vi "VISA_ReadAndSave_8CHparalelos.vi"() -> ()   [LabVIEW 2019]
uses:
  813f916b-c519-439e-9418-14bd48b6d342.vi
  <vilib>/Instr/_visa.llb/VISA Configure Serial Port (Instr).vi
  <vilib>/Analysis/Matrix/Comparison/Not Equal/Not Equal.vi
  <vilib>/Analysis/Matrix/Comparison/Not Equal/Not Equal - RM,RM.vi
panel:
  out "loop delay":dbl format="%.2f"
  out "Plot 7":dbl[](graph)
  out "Plot 6":dbl[](graph)
  out "Plot 5":dbl[](graph)
  out "Plot 4":dbl[](graph)
  out "Plot 3":dbl[](graph)
  out "Plot 2":dbl[](graph)
  out "error file":errorcluster
  in  "file name":string
  out "Plot 1":dbl[](graph)
  out "Plot 0":dbl[](graph)
  out "Status Read":errorcluster
  out "Buffer Array":dbl[](array[numeric])
  out "Read Buffer":string
  out "Status Serial":errorcluster
  in  "Stop Read":bool
  in  "Start Read":bool
  in  "baud rate (115200)":u32=115200 caption="baud rate (9600)"
  in  "data bits (8)":u8=8 min=5 max=8 step=1
  in  "VISA resource name":refnum<visa-resource-name>="COM3"
  # "Controle de Salvamento"
  # "Log de Erros"
  # "Conversão Para Inteiro"
  # "Resultado da Leitura"
  # "Controle da porta Serial USB"
  # "Controle da Leitura"
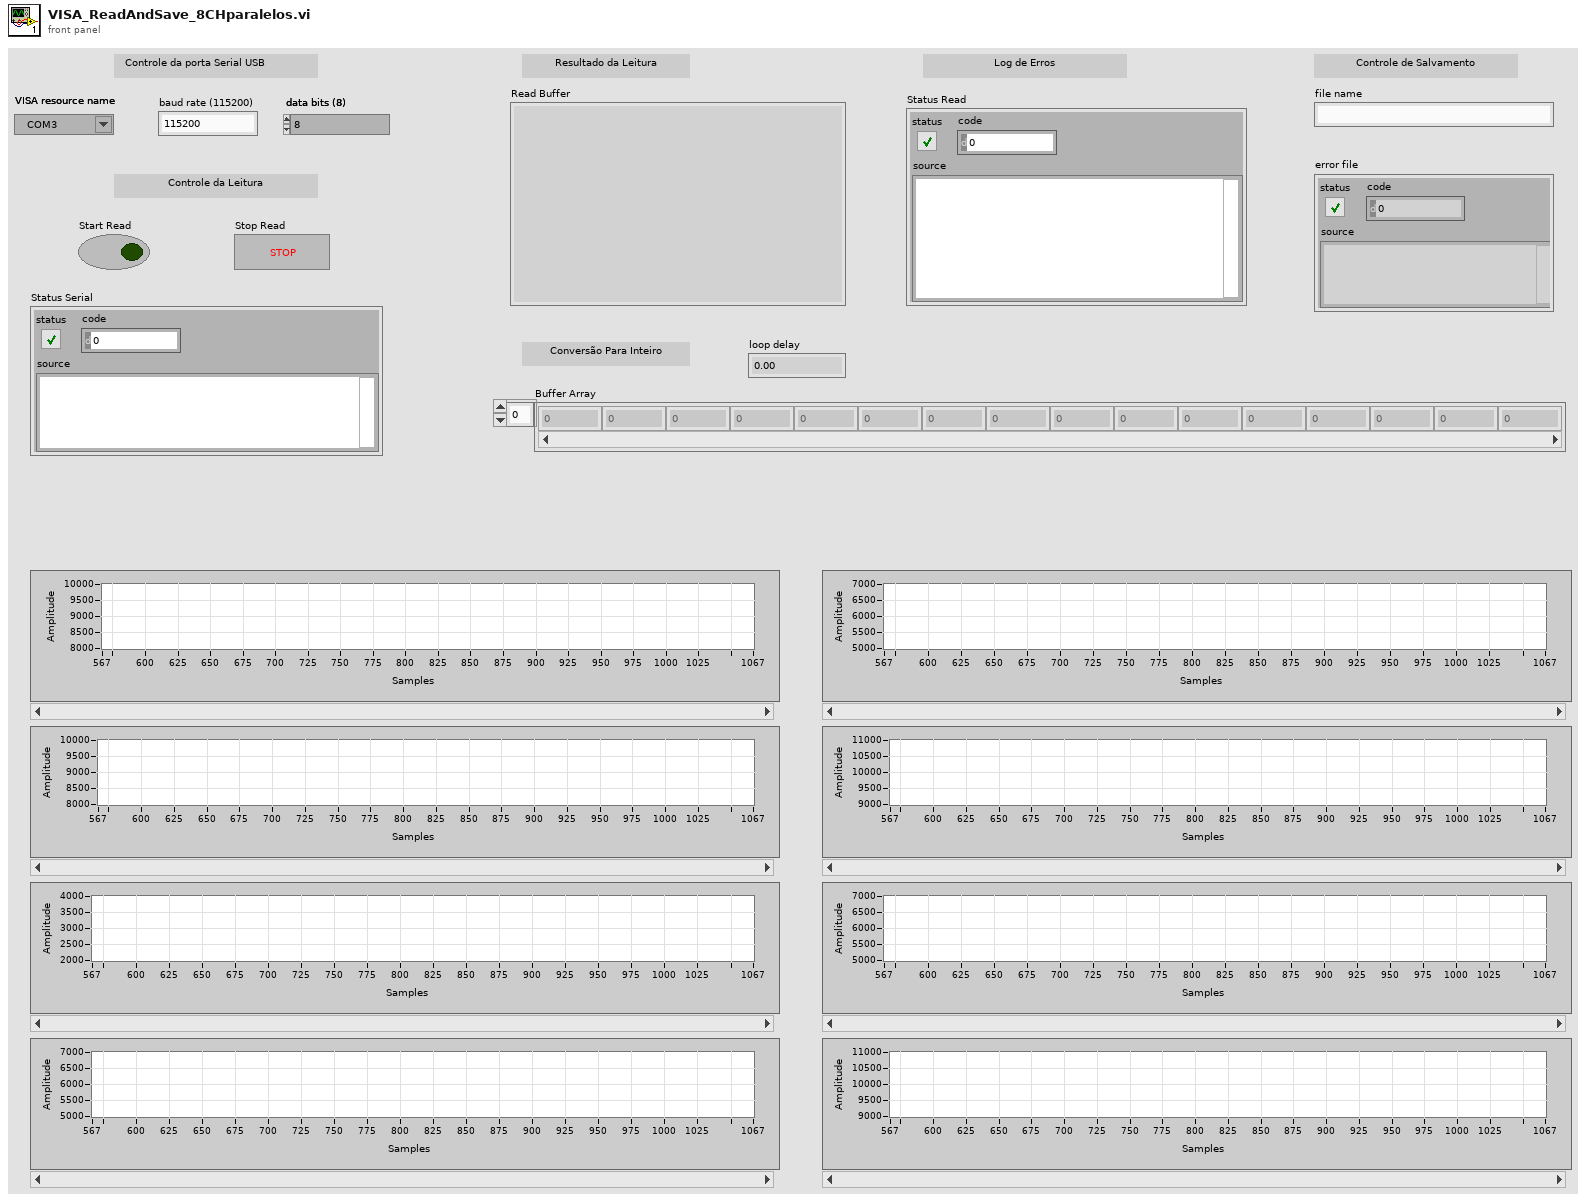
[diagram p1: front panel]
types:
  T1 = typedef "NI_Matrix.lvlib/RealMatrix.ctl" = dbl[][]
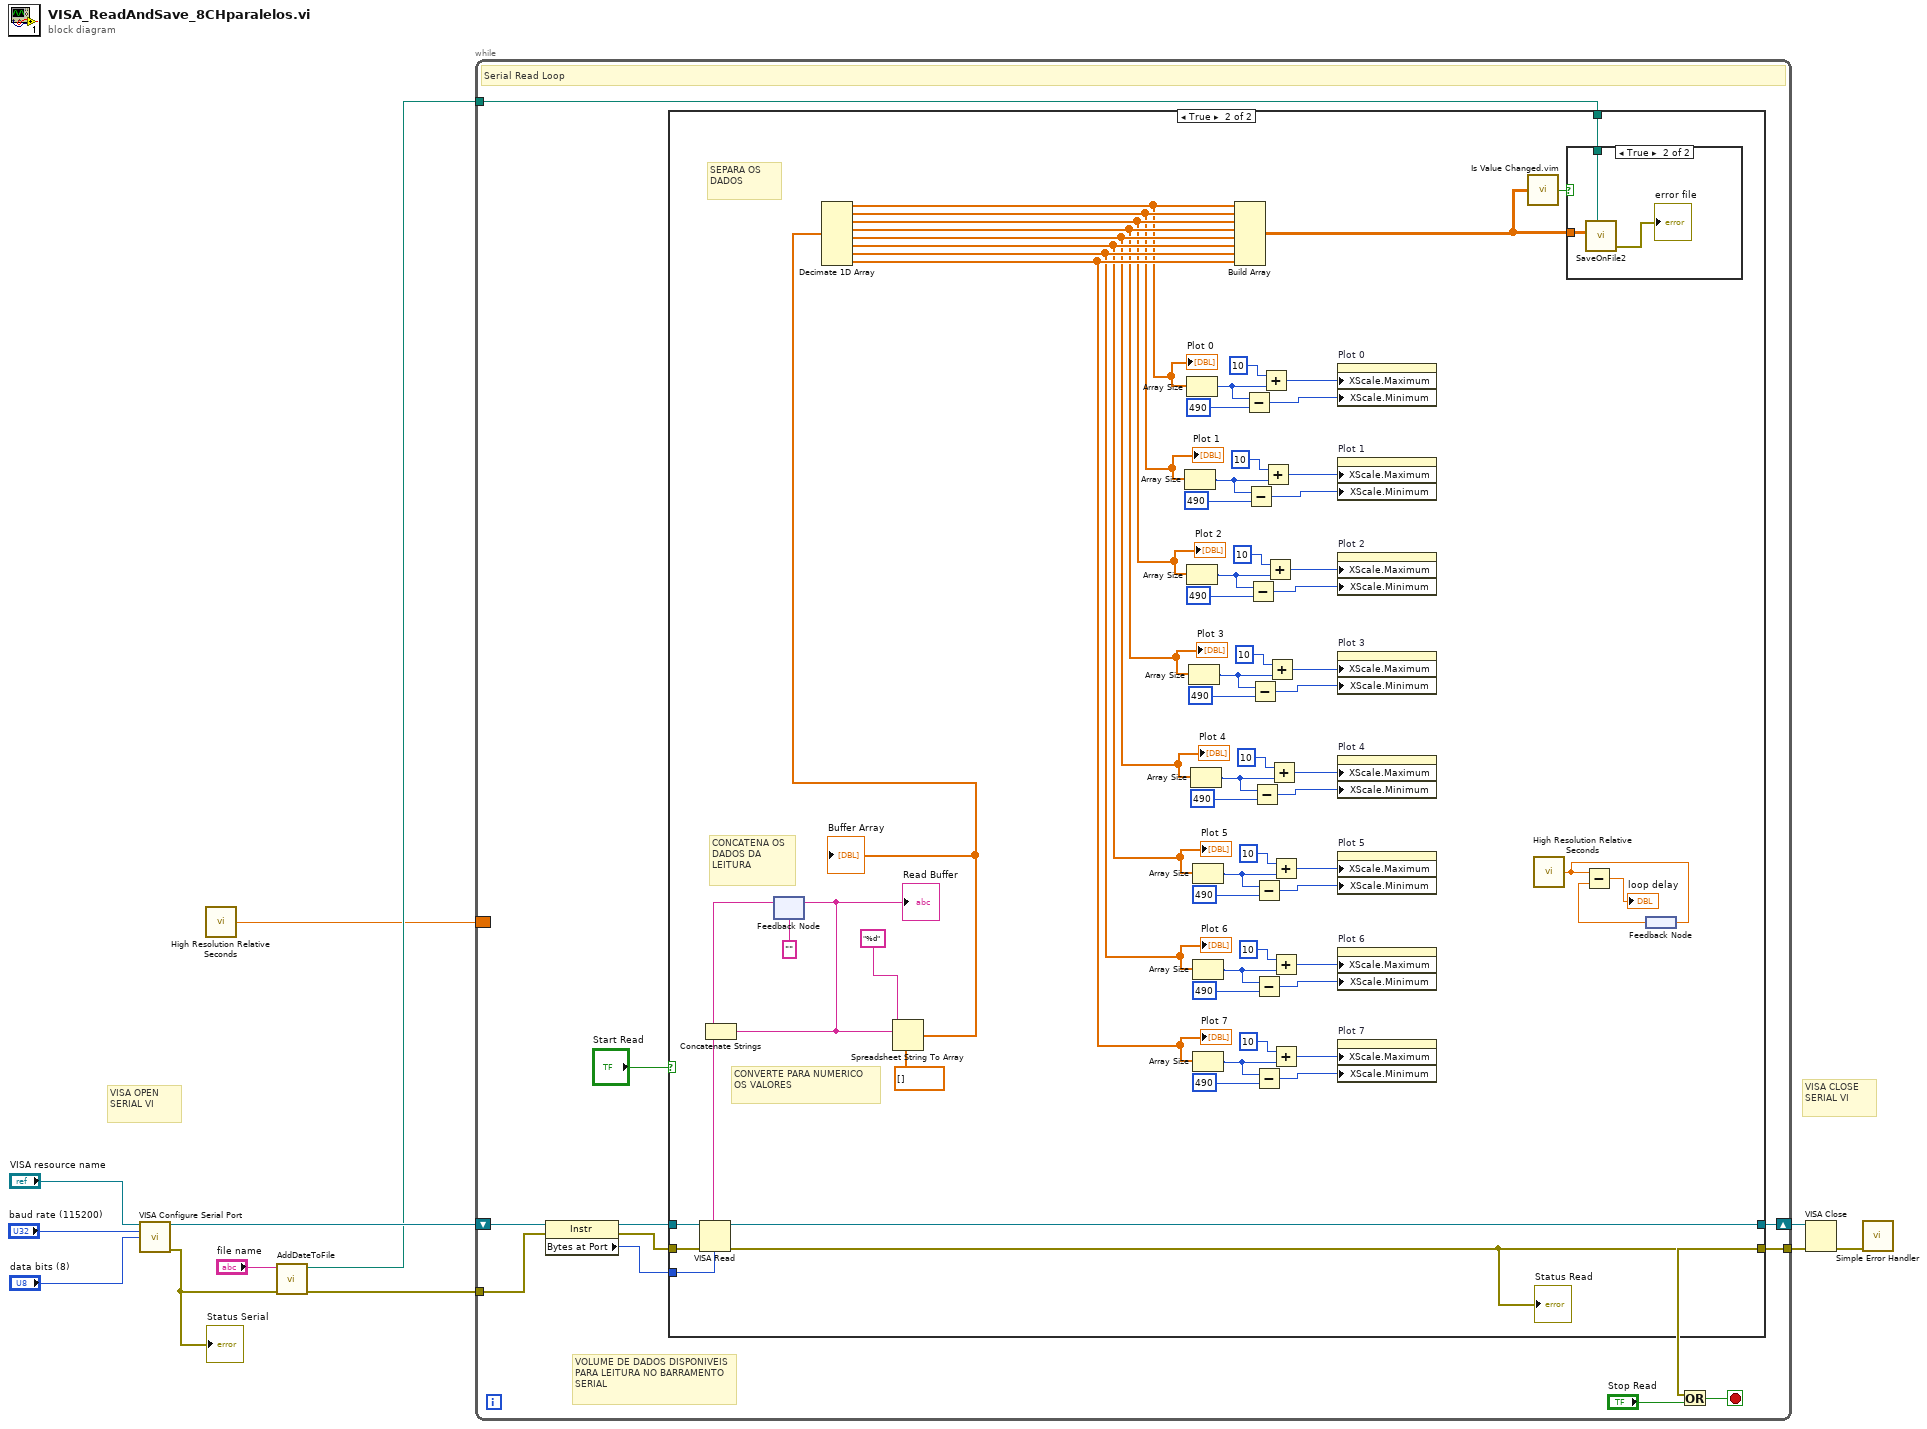
[diagram p0: block diagram]
diagram:
  # "VISA OPEN SERIAL VI"
  # "VISA CLOSE SERIAL VI"
  n1 = call-poly "VISA Configure Serial Port"("VISA resource name"="VISA resource name", "baud rate (9600)"="baud rate (115200)", "data bits (8)"="data bits (8)") -> ("VISA resource name out"=w10:refnum<visa-resource-name>, "error out"=w3:errorcluster)  [unwired: 11 in]
  "Status Serial" <- w3
  n2 = call <vilib>:"High Resolution Relative Seconds.vi"() -> ("relative seconds"=w1:dbl)
  n3 = call "AddDateToFile.vi"("error in (no error)"=w3, "file name"="file name") -> ("error out"=w4:errorcluster, "new file path (Not A Path if cancelled)"=w2:path)  [unwired: 8 in]
  n4 = while {
    tunnel: w4 -> [w14]
    tunnel: [w21] -> w11
    shift-right: [w20] -> w9
    shift-left: w10 -> [w18]
    tunnel: w2 -> [w13]
    border: w1 -> [_]
    stop <- w19 stop-if-true
    # "VOLUME DE DADOS DISPONIVEIS PARA LEITURA NO BARRAMENTO SERIAL"
    # "Serial Read Loop"
    n5 = property class="Instr"(reference=w18, error in=w14) -> (reference out=w15:refnum<visa-resource-name>, error out=w16:errorcluster, "Bytes at Port"=w17:u32)
    n6 = case shown="True" "Start Read" {
      tunnel: [w24 w91] -> w21
      tunnel: [w25 w89] -> w20
      tunnel: w17 -> [_ w85]
      tunnel: w15 -> [w25 w84]
      tunnel: w16 -> [w24 w83]
      tunnel: w13 -> [_ w75]
      frame False {
        # "OS DADOS SÃO ACUMULADOS NO BUFFER ESPERANDO A PERMISSÃO PARA SER LIDOS"
      }
      frame True {
        # "SEPARA OS DADOS"
        # "CONVERTE PARA NUMERICO OS VALORES"
        # "CONCATENA OS DADOS DA LEITURA"
        n7 = VISA Read(VISA resource name=w84, byte count=w85, error in (no error)=w83) -> (VISA resource name out=w89:refnum<visa-resource-name>, read buffer=w39:string, error out=w91:errorcluster)  [unwired: 1 out]
        "Status Read" <- w91
        n8 = feedback #1("") -> (w86:string)
        n9 = Concatenate Strings(w86, w39) -> (w88:string)
        "Read Buffer" <- w88
        n10 = feedback-in #1(w88) -> ()
        n11 = Spreadsheet String To Array(format string="%d", spreadsheet string=w88, array type (2D Dbl)=dbl[] []) -> (array=w38:dbl[])  [unwired: 1 in]
        "Buffer Array" <- w38
        n12 = Decimate 1D Array(w38) -> (w26:dbl[], w27:dbl[], w28:dbl[], w29:dbl[], w30:dbl[], w31:dbl[], w32:dbl[], w33:dbl[])
        "Plot 0" <- w26
        "Plot 1" <- w27
        "Plot 2" <- w28
        "Plot 3" <- w29
        "Plot 4" <- w30
        "Plot 5" <- w31
        "Plot 6" <- w32
        "Plot 7" <- w33
        n13 = Array Size(array=w27) -> (size(s)=w71:i32)
        n14 = Array Size(array=w26) -> (size(s)=w78:i32)
        n15 = Array Size(array=w28) -> (size(s)=w68:i32)
        n16 = Array Size(array=w29) -> (size(s)=w65:i32)
        n17 = Array Size(array=w30) -> (size(s)=w62:i32)
        n18 = Array Size(array=w31) -> (size(s)=w59:i32)
        n19 = Array Size(array=w32) -> (size(s)=w56:i32)
        n20 = Array Size(array=w33) -> (size(s)=w53:i32)
        n21 = Build Array(w26, w27, w28, w29, w30, w31, w32, w33) -> (w37:T1)
        n22 = Subtract(x=w78, y=490) -> (x-y=w79:i32)
        n23 = Subtract(x=w71, y=490) -> (x-y=w74:i32)
        n24 = Subtract(x=w68, y=490) -> (x-y=w50:i32)
        n25 = Subtract(x=w65, y=490) -> (x-y=w48:i32)
        n26 = Subtract(x=w62, y=490) -> (x-y=w43:i32)
        n27 = Subtract(x=w59, y=490) -> (x-y=w42:i32)
        n28 = Subtract(x=w56, y=490) -> (x-y=w41:i32)
        n29 = Subtract(x=w53, y=490) -> (x-y=w40:i32)
        n30 = Add(x=10, y=w78) -> (x+y=w77:i32)
        n31 = Add(x=10, y=w71) -> (x+y=w73:i32)
        n32 = Add(x=10, y=w68) -> (x+y=w51:i32)
        n33 = Add(x=10, y=w65) -> (x+y=w49:i32)
        n34 = Add(x=10, y=w62) -> (x+y=w47:i32)
        n35 = Add(x=10, y=w59) -> (x+y=w46:i32)
        n36 = Add(x=10, y=w56) -> (x+y=w45:i32)
        n37 = Add(x=10, y=w53) -> (x+y=w44:i32)
        n38 = property on="Plot 0" class="WFGraph (strict)"("XScale.Maximum"=w77, "XScale.Minimum"=w79) -> ()  [unwired: 2 in, 2 out]
        n39 = property on="Plot 1" class="WFGraph (strict)"("XScale.Maximum"=w73, "XScale.Minimum"=w74) -> ()  [unwired: 2 in, 2 out]
        n40 = property on="Plot 2" class="WFGraph (strict)"("XScale.Maximum"=w51, "XScale.Minimum"=w50) -> ()  [unwired: 2 in, 2 out]
        n41 = property on="Plot 3" class="WFGraph (strict)"("XScale.Maximum"=w49, "XScale.Minimum"=w48) -> ()  [unwired: 2 in, 2 out]
        n42 = property on="Plot 4" class="WFGraph (strict)"("XScale.Maximum"=w47, "XScale.Minimum"=w43) -> ()  [unwired: 2 in, 2 out]
        n43 = property on="Plot 5" class="WFGraph (strict)"("XScale.Maximum"=w46, "XScale.Minimum"=w42) -> ()  [unwired: 2 in, 2 out]
        n44 = property on="Plot 6" class="WFGraph (strict)"("XScale.Maximum"=w45, "XScale.Minimum"=w41) -> ()  [unwired: 2 in, 2 out]
        n45 = property on="Plot 7" class="WFGraph (strict)"("XScale.Maximum"=w44, "XScale.Minimum"=w40) -> ()  [unwired: 2 in, 2 out]
        n46 = call "Is Value Changed.vim"("value"=w37) -> ("changed or first call?"=w81:bool)
        n47 = call <vilib>:"High Resolution Relative Seconds.vi"() -> ("relative seconds"=w35:dbl)
        n48 = case shown="True" w81 {
          tunnel: w37 -> [_ w92]
          tunnel: w75 -> [_ w94]
          frame False {
          }
          frame True {
            n49 = call "SaveOnFile2.vi"("2D data"=w92, "file path (dialog if empty)"=w94) -> ("error file"=→"error file":errorcluster)  [unwired: 5 in]
          }
        }
        n50 = feedback #2() -> (w36:dbl)
        n51 = Subtract(x=w35, y=w36) -> (x-y=→"loop delay":dbl)
        n52 = feedback-in #2(w35) -> ()
      }
    }
    n53 = Or(x=w21, y="Stop Read") -> (x .or. y?=w19:bool)
  }
  n54 = VISA Close(VISA resource name=w9, error in (no error)=w11) -> (error out=w8:errorcluster)
  n55 = call <vilib>:"Simple Error Handler.vi"("error in (no error)"=w8) -> ()  [unwired: 4 in, 5 out]
